vi "WaveGenerator_Sample_Program.vi"(0 "System no.":i32=1 min=1 max=4 step=1, 1 "Stop refnum":refnum<vi>, 2 "Affected axis":string="1", 3 "Selection":T1, 4 "DDL":bool, 5 "error in":errorcluster, 6 "Sine Parameters:":T3={"Xo (Start)"=0, "SIN_P Parameters"={"C"=200.0, "A"=10.0, "O"=0.0}, "N (Length)"=500, "Append? (&)"=FALSE} {"N (Length)" min=0 max=1000 step=1; "SIN_P Parameters"."O" format="%.6f"; "SIN_P Parameters"."A" format="%.6f"; "SIN_P Parameters"."C" format="%.6f"}, 7 "Ramp Parameters:":T2={"Xo (Start)"=0, "RAMP Parameters"={"C"=200.0, "J"=0.0, "A"=8.0, "O"=0.0}, "N (Length)"=500, "Append? (&)"=FALSE} {"N (Length)" min=0 max=1000 step=1; "RAMP Parameters"."O" format="%.6f"; "RAMP Parameters"."A" format="%.6f"; "RAMP Parameters"."J" format="%.6f"; "RAMP Parameters"."C" format="%.6f"}, 8 "Start position":dbl format="%.6f") -> (14 "Waveform":dbl[][](graph) caption="Graph showing the commanded (green) and measured (white) waveform and the position error (red).", 19 "Error out":errorcluster)   [LabVIEW 2009]
doc: "This VI demonstrates how to use the wave generator command VIs. It first moves the affected axis to a given start position. Then it runs in a loop, giving the user the options to write sine wave curve segments or ramps into the controllers wave buffer. Wave storage data points are limited to 1000 points to keep transfer times low. The segment length of one waveform - which normally defines the frequency - is predefined as 500 points in this example. Depending on the value of Append? (&), either the old buffer data is overwritten or the new wave will be appended to memory. Please take into account that you can append at most two waveforms since buffer size is limited to 1000 points as mentioned above. \n\nAdjust the following controls to modify the shape of the waveforms.\nN (Length): Waveform (i.e. the points to be modified) goes from 1 to Length. Datapoints from Length to 500 are filled with value of last wave point.\nXo (Start): Position where the first point of the waveform is located. \nC: Center point of the wave. If C = Length/2 then the wave is symmetrical.\nA: Amplitude of the waveform. F(x) = A*sin(x) + O\nO: Offset of the waveform. F(x) = A*sin(x) + O\nJ: Jerk. Means curvature in the transition to or from standstill.\n\nYou have to stop generator output prior to restarting it with a different parameter set. The Start Gen. and Stop Gen. buttons will enable or disable the wave generator output by sending \"WGO 0\" or \"WGO 1\" for the affected axis. If DDL is enabled \"WGO 65\" will be sent respectively. The red Stop button stops the wave generator output on the specified axis and finishes the loop. Please respect the delays that occur while the controller is processing your commands. This is indicated by the \"Busy?\" indicator. See manual for further details. \n\nIn case of an error a button Clear Error will appear and the control buttons above will be disabled. Pressing this button will clear the error status and enable the control buttons again.\nWith DDL ON you can achieve significantly better position accuracy. Compare the target (green), response (white) and error (red) signals on the graph. Since this is a very sensitive mechanism we recommend starting with low amplitudes and adjusting the parameters with caution. The DDL button works only if the controller supports DDL. Contact PI for information on activation of DDL support.\n\nSee User Manual for details about the use of the wave generator.\n\nRun XXXX_Configuration_Setup (with XXXX being the product number of your PI controller) prior to running this VI.\n\nValid for: E-753"
panel:
  out "Gen. running?":bool
  out "DDL":bool
  in  "Clear Error":bool
  out "Busy?":bool
  out "Controller error":bool
  in  "Stop":bool
  # "Wave generator sample program"
  # "This VI demonstrates how to use the wave generator command VIs. It first moves the affected axis to a given start position. Then it runs in a loop, giving the\nuser the options to write sine wave curve segments or ramps into the controllers wave buffer. Wave storage data points are limited to 1000 points\nto keep transfer times low. The segment length of one waveform is predefined as 500 points in this example. Depending on the value of Append? (&), either\nthe old buffer data is overwritten or the new wave will be appended to memory. You have to stop generator output prior to restarting it with a different\nparameter set. The Start Gen. and Stop Gen. buttons will enable or disable the wave generator output by sending \"WGO 0\" or \"WGO 1\" for the affected axis. \nIf DDL is enabled \"WGO 65\" will be sent respectively. The red Stop button stops the wave generator output on the specified axis and finishes the loop. Please\nrespect the delays that occur while the controller is processing your commands. This is indicated by the \"Busy?\" indicator. See manual for further details. \nRun XXXX_Configuration_Setup (with XXXX being the product number of your PI controller) prior to running this VI."
  # "DDL state"
  # "Stop VI\nand wave\ngenerator\noutput"
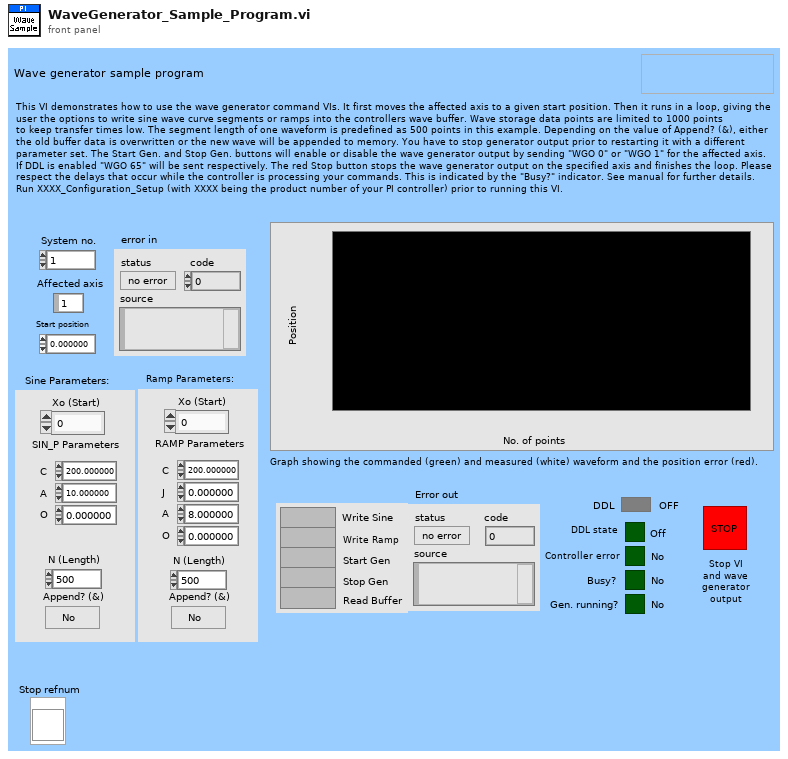
[diagram p1: front panel]
types:
  T1 = cluster{"Write Sine":bool, "Write Ramp":bool, "Start Gen":bool, "Stop Gen":bool, "Read Buffer":bool}
  T2 = cluster{"Xo (Start)":i32, "RAMP Parameters":cluster{"C":dbl, "J":dbl, "A":dbl, "O":dbl}, "N (Length)":i32, "Append? (&)":bool}
  T3 = cluster{"Xo (Start)":i32, "SIN_P Parameters":cluster{"C":dbl, "A":dbl, "O":dbl}, "N (Length)":i32, "Append? (&)":bool}
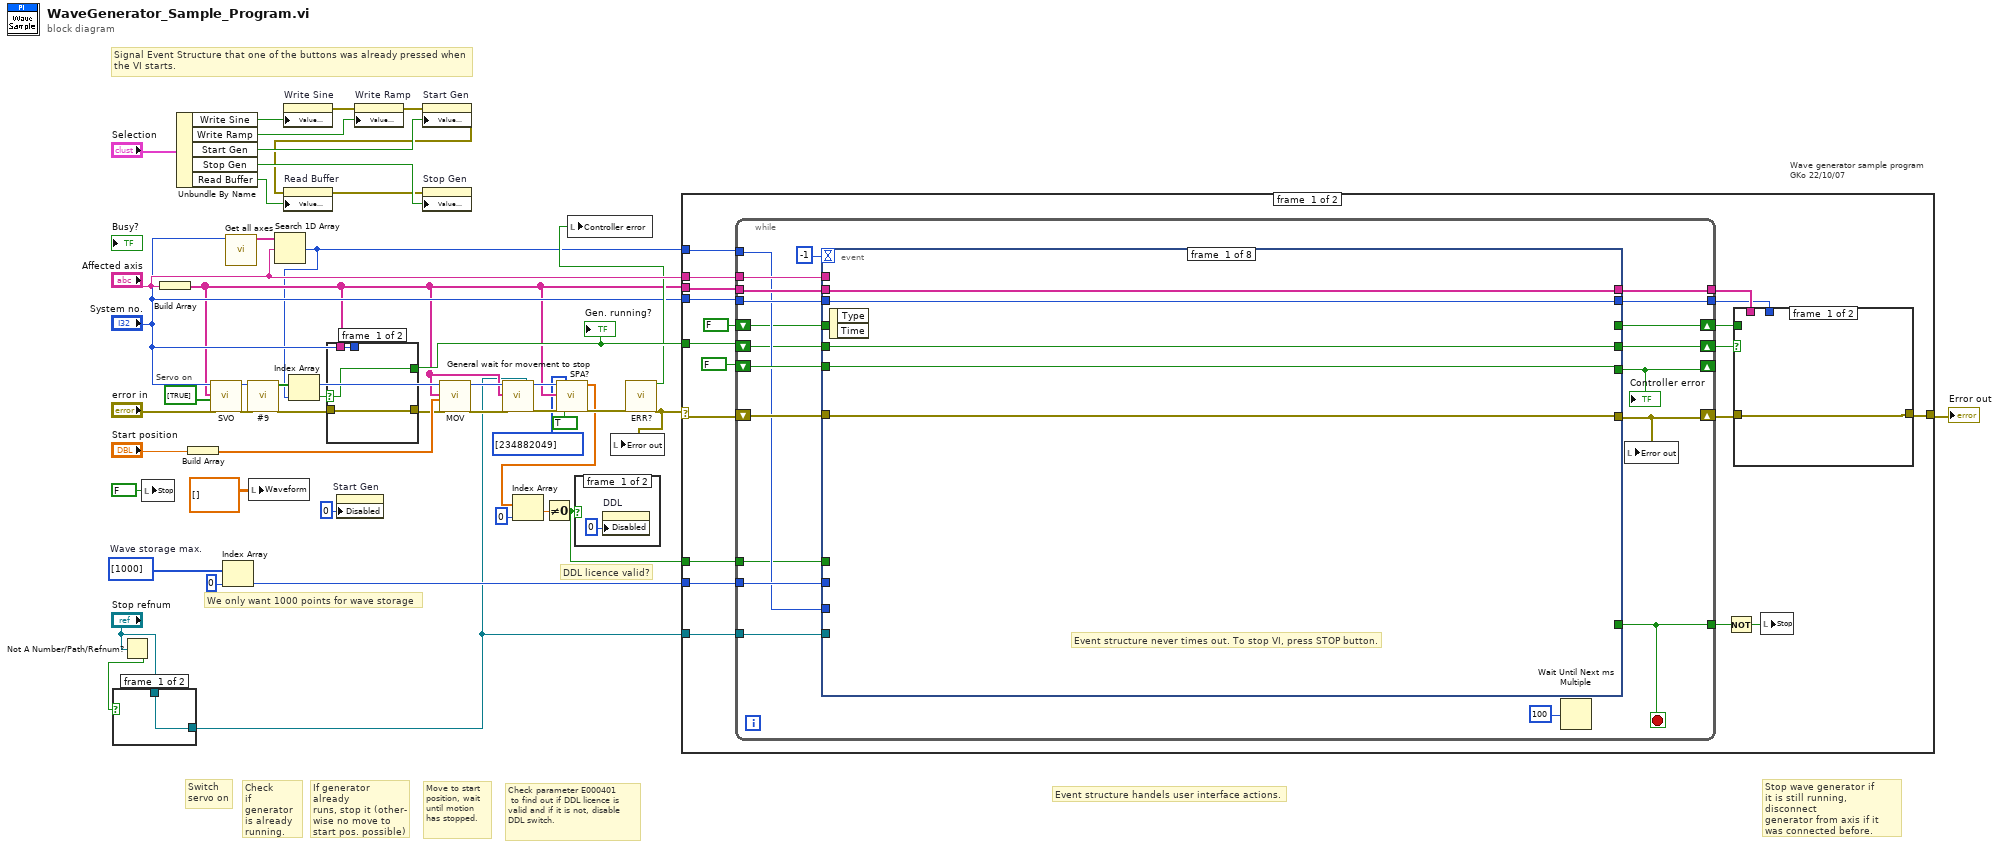
[diagram p0: block diagram]
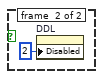
[diagram p2: hidden frame]
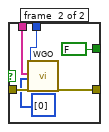
[diagram p3: hidden frame]
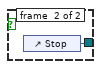
[diagram p4: hidden frame]
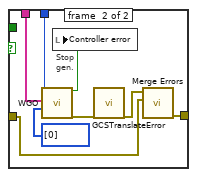
[diagram p5: hidden frame]
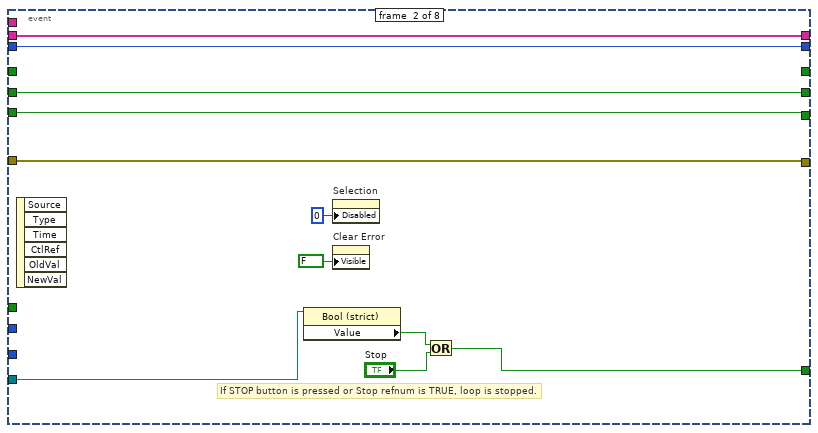
[diagram p6: hidden frame]
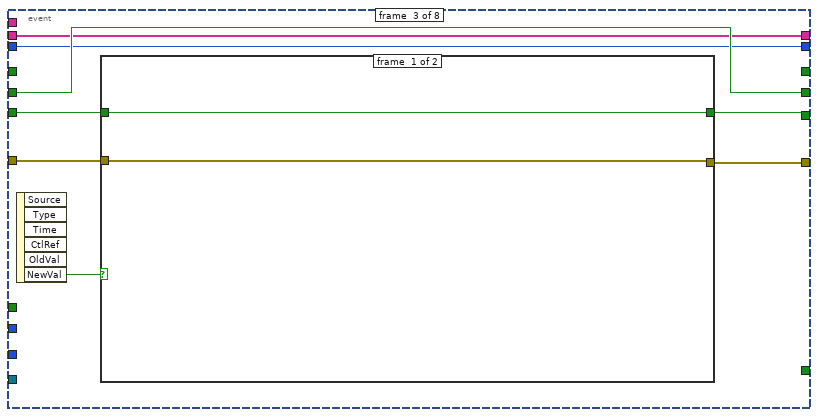
[diagram p7: hidden frame]
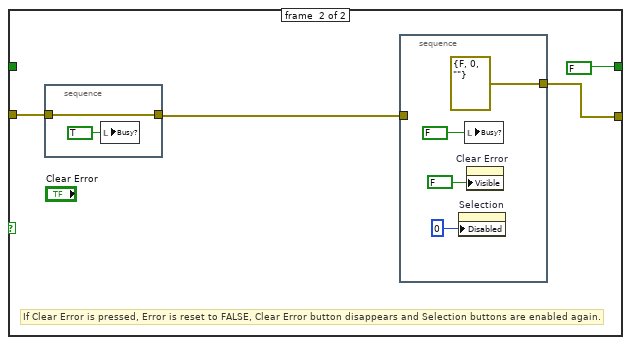
[diagram p8: hidden frame]
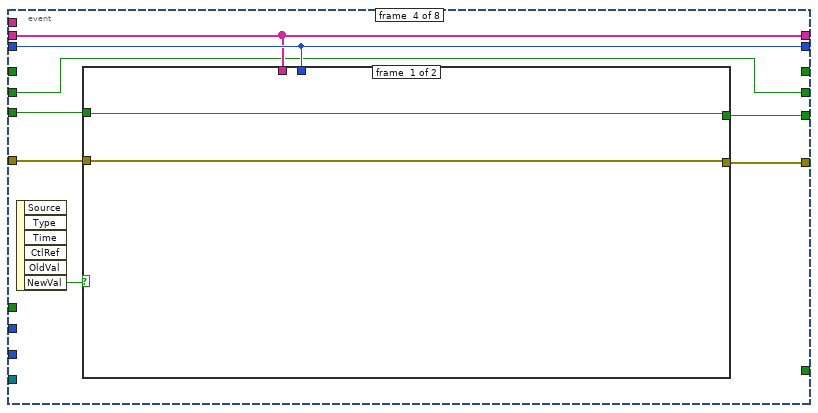
[diagram p9: hidden frame]
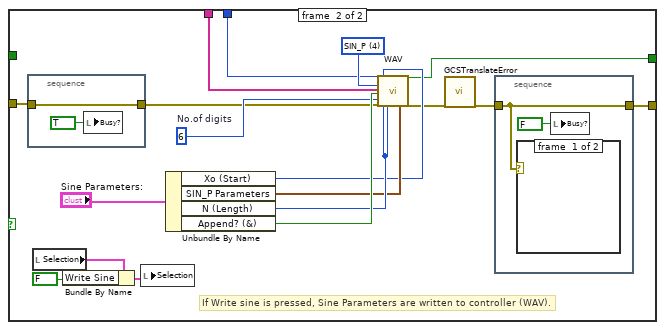
[diagram p10: hidden frame]
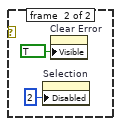
[diagram p11: hidden frame]
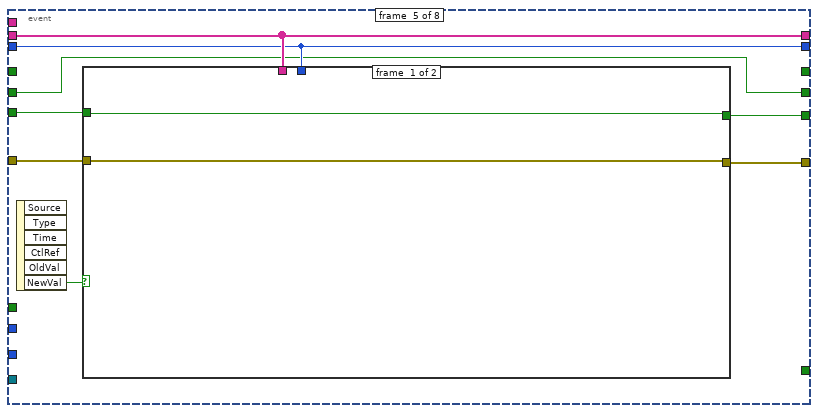
[diagram p12: hidden frame]
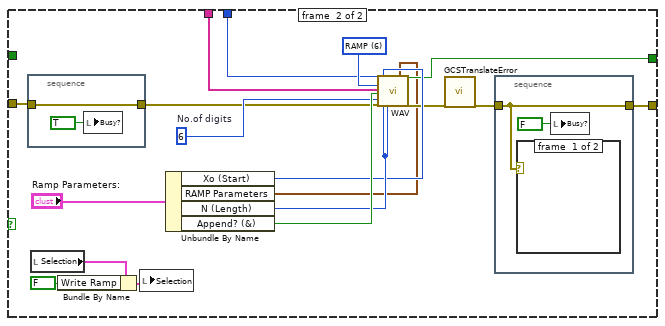
[diagram p13: hidden frame]
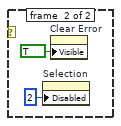
[diagram p14: hidden frame]
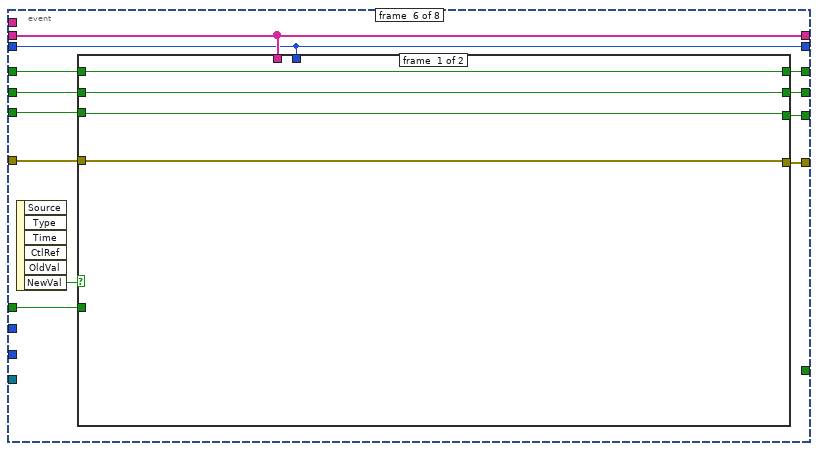
[diagram p15: hidden frame]
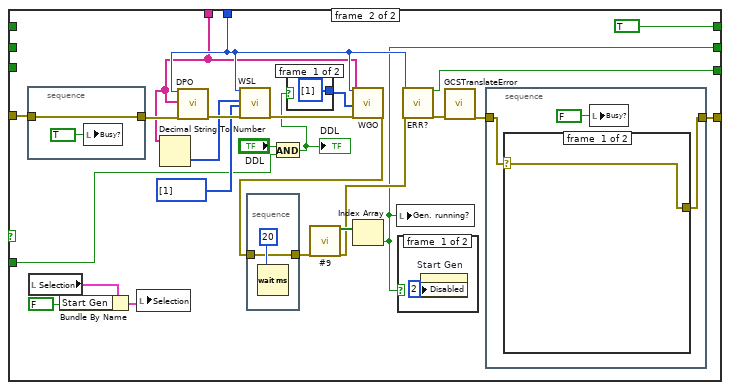
[diagram p16: hidden frame]
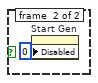
[diagram p17: hidden frame]
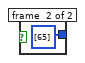
[diagram p18: hidden frame]
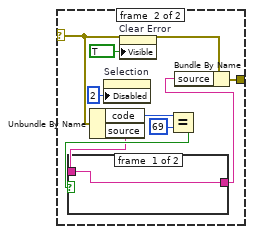
[diagram p19: hidden frame]
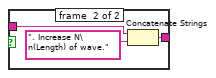
[diagram p20: hidden frame]
diagram:
  w43 = i32[] [1000]  # Wave storage max.
  # "Stop wave generator if\nit is still running, disconnect \ngenerator from axis if it\nwas connected before."
  # "Event structure handels user interface actions."
  # "Check parameter E000401\n to find out if DDL licence is\nvalid and if it is not, disable\nDDL switch."
  # "If generator already\nruns, stop it (other-\nwise no move to\nstart pos. possible)"
  # "Check\nif generator\nis already \nrunning."
  # "We only want 1000 points for wave storage"
  # "Switch\nservo on"
  # "Signal Event Structure that one of the buttons was already pressed when\nthe VI starts."
  # "DDL licence valid?"
  # "Servo on"
  # "Move to start\nposition, wait\nuntil motion\nhas stopped."
  # "Wave generator sample program\nGKo 22/10/07"
  n1 = Not A Number/Path/Refnum?(number/path/refnum="Stop refnum") -> (NaN/Path/Refnum?=w39:bool)
  n2 = case shown="True" w39 {
    tunnel: [w47 w48] -> w5
    tunnel: "Stop refnum" -> [w47 _]
    frame #0 {
    }
    frame #1 {
      n3 = control-ref of="Stop"() -> (w48:refnum<vi>)
    }
  }
  n4 = local write "Stop"(FALSE ("Controller error")) -> ()
  n5 = Build Array("Affected axis") -> (w19:string[])
  n6 = Unbundle By Name("Selection") -> ("Write Sine"=w10:bool, "Write Ramp"=w9:bool, "Start Gen"=w8:bool, "Stop Gen"=w7:bool, "Read Buffer"=w6:bool)
  n7 = Build Array("Start position") -> (w40:dbl[])
  n8 = call "SVO.vi"("System no."="System no.", "Axes to command"=w19, "Servo mode"=bool[] [TRUE], "error in"="error in") -> ("error out"=w33:errorcluster)  [unwired: 15 in]
  n9 = Index Array(array=w43, index=0 ("Index")) -> (element=w44:i32)
  n10 = call "Get all axes.vi"("System no."="System no.") -> ("Conn. Axes"=w35:string[])  [unwired: 18 in]
  n11 = call "#9.vi"("System no."="System no.", "error in"=w33) -> ("WG running?"=w36:bool[], "error out"=w28:errorcluster)  [unwired: 16 in]
  n12 = local write "Waveform"(dbl[][] [] ("Waveform")) -> ()
  n13 = Search 1D Array(1D array=w35, element="Affected axis") -> (index of element=w15:i32)  [unwired: 1 in]
  n14 = property on="Write Sine" class="Boolean (strict)"("Value (Signaling)"=w10) -> (error out=w4:errorcluster)  [unwired: 2 in, 1 out]
  n15 = Index Array(array=w36, index=w15) -> (element=w29:bool)
  n16 = case shown="True" w29 {
    selector: w29 -> [w50 _]
    tunnel: w28 -> [w49 w56]
    tunnel: [w49 w55] -> w27
    tunnel: "System no." -> [_ w53]
    tunnel: w19 -> [_ w52]
    tunnel: [w50 FALSE] -> w26
    frame #0 {
    }
    frame #1 {
      n17 = call "WGO.vi"("System no."=w53, "Affected axes"=w52, "WGO Parameter"=i32[] [0], "error in"=w56) -> ("error out"=w55:errorcluster)  [unwired: 14 in, 1 out]
    }
  }
  "Gen. running?" <- w26
  n18 = property on="Start Gen" class="Bool (strict)"("Disabled"=u8 0) -> ()  [unwired: 2 in, 2 out]
  n19 = property on="Write Ramp" class="Boolean (strict)"(error in=w4, "Value (Signaling)"=w9) -> (error out=w3:errorcluster)  [unwired: 1 in, 1 out]
  n20 = property on="Start Gen" class="Boolean (strict)"(error in=w3, "Value (Signaling)"=w8) -> (error out=w2:errorcluster)  [unwired: 1 in, 1 out]
  n21 = property on="Stop Gen" class="Boolean (strict)"(error in=w2, "Value (Signaling)"=w7) -> (error out=w1:errorcluster)  [unwired: 1 in, 1 out]
  n22 = property on="Read Buffer" class="Boolean (strict)"(error in=w1, "Value (Signaling)"=w6) -> ()  [unwired: 1 in, 2 out]
  n23 = call "MOV.vi"("System no."="System no.", "Axes to move"=w19, "Position values"=w40, "error in"=w27) -> ("error out"=w30:errorcluster)  [unwired: 15 in]
  n24 = call "General wait for movement to stop.vi"("System no."="System no.", "Axes to wait for"=w19, "error in"=w30, "Stop refnum"=w5) -> ("error out"=w21:errorcluster)  [unwired: 14 in, 1 out]
  n25 = call "SPA?.vi"("System no."="System no.", "Axes to query"=w19, "error in"=w21, "Parameter no. (hex)"=u32[] [234882049], "Parameter no. format \n(Decimal: FALSE)"=TRUE ("Parameter no. format \n(Decimal: FALSE)")) -> ("Parameter value"=w16:dbl[], "error out"=w22:errorcluster)  [unwired: 9 in, 4 out]
  n26 = Index Array(array=w16, index=0) -> (element=w13:dbl)
  n27 = Not Equal To 0?(x=w13) -> (x != 0?=w12:bool)
  n28 = case shown="True" w12 {
    frame #0 {
      n29 = property on="DDL" class="Boolean (strict)"("Disabled"=u8 0) -> ()  [unwired: 2 in, 2 out]
    }
    frame #1 {
      n30 = property on="DDL" class="Boolean (strict)"("Disabled"=u8 2) -> ()  [unwired: 2 in, 2 out]
    }
  }
  n31 = call "ERR?.vi"("error in"=w22) -> ("Controller error"=w24:bool, "error out"=w25:errorcluster)  [unwired: 17 in]
  n32 = local write "Controller error"(w24) -> ()
  n33 = local write "Error out"(w25) -> ()
  n34 = case shown="No Error" w25 {
    selector: w25 -> [w69 w372]
    tunnel: w19 -> [w77 _]
    tunnel: "System no." -> [w76 _]
    tunnel: [w67 w371] -> w46
    tunnel: w44 -> [w70 _]
    tunnel: "Affected axis" -> [w72 _]
    tunnel: w15 -> [w68 _]
    tunnel: w26 -> [w66 _]
    tunnel: w12 -> [w60 _]
    tunnel: w5 -> [w59 _]
    frame #0 {
      n35 = while {
        tunnel: w72 -> [w98]
        tunnel: w70 -> [w99]
        shift-left: w69 -> [w101]
        shift-right: [w100] -> w73
        tunnel: [w102] -> w74
        tunnel: [w104] -> w75
        tunnel: w76 -> [w103]
        tunnel: w77 -> [w105]
        shift-right: [w96] -> _
        shift-left: FALSE ("Controller error") -> [w95]
        tunnel: w68 -> [w94]
        shift-right: [w92] -> w65
        shift-left: w66 -> [w93]
        tunnel: [w91] -> w64
        shift-right: [w90] -> w61
        shift-left: FALSE -> [w89]
        tunnel: w60 -> [w88]
        tunnel: w59 -> [w87]
        stop <- w91 stop-if-true
        n36 = event shown="[4] \"Selection.Write Ramp\": Value Change" {
          selector: _ -> [_ _ _ _ _ _ _ _]
          dyn-events: _ -> [_ _ _ _ _ _ _ _]
          timeout: -1 -> [_ _ _ _ _ _ _ _]
          tunnel: w105 -> [w109 w120 w123 w144 w179 w217 w280 w319]
          tunnel: [w109 w120 w123 w144 w179 w217 w280 w319] -> w104
          tunnel: w103 -> [w108 w119 w124 w145 w178 w216 w279 w320]
          tunnel: [w108 w119 w124 w145 w178 w216 w279 w320] -> w102
          tunnel: w101 -> [w110 w121 w126 w148 w182 w220 w284 w326]
          tunnel: [w110 w121 w127 w149 w183 w221 w285 w327] -> w100
          tunnel: w99 -> [_ _ _ _ _ _ _ w321]
          tunnel: w98 -> [_ _ _ _ _ _ _ w322]
          tunnel: [w111 w122 w128 w150 w184 w222 w286 w328] -> w96
          tunnel: w95 -> [w111 w122 w129 w146 w180 w218 w282 w324]
          tunnel: w94 -> [_ _ _ _ _ _ w281 w323]
          tunnel: [_ w114 _ _ _ _ _ _] -> w91
          tunnel: w93 -> [w107 w118 w125 w143 w177 w214 w277 w318]
          tunnel: [w107 w118 w125 w143 w177 w215 w278 w318] -> w92
          tunnel: [_ _ _ _ _ w213 _ _] -> w90
          tunnel: w89 -> [_ _ _ _ _ w212 _ _]
          tunnel: w88 -> [_ _ _ _ _ w211 _ _]
          tunnel: w87 -> [_ w117 _ _ _ _ _ _]
          event #0 {
            # "Event structure never times out. To stop VI, press STOP button."
            n37 = event-data() -> ()  [unwired: 1 in, 2 out]
          }
          event #1 {
            # "If STOP button is pressed or Stop refnum is TRUE, loop is stopped."
            n38 = event-data() -> ()  [unwired: 1 in, 6 out]
            n39 = property class="Bool (strict)"(reference=w117) -> ("Value"=w116:bool)  [unwired: 1 in, 2 out]
            n40 = property on="Selection" class="Cluster (strict)"("Disabled"=u8 0) -> ()  [unwired: 2 in, 2 out]
            n41 = property on="Clear Error" class="Boolean"("Visible"=FALSE) -> ()  [unwired: 2 in, 2 out]
            n42 = Or(x=w116, y="Stop") -> (x .or. y?=w114:bool)
          }
          event #2 {
            n43 = event-data() -> ("NewVal"=w130:bool)  [unwired: 1 in, 5 out]
            n44 = case shown="True" w130 {
              tunnel: w129 -> [w132 _]
              tunnel: [w132 FALSE ("Controller error")] -> w128
              tunnel: [w131 w134] -> w127
              tunnel: w126 -> [w131 w135]
              frame #0 {
              }
              frame #1 {
                # "If Clear Error is pressed, Error is reset to FALSE, Clear Error button disappears and Selection buttons are enabled again."
                n45 = stacked-sequence {
                  tunnel: w135 -> [w141]
                  tunnel: [w141] -> w133
                  frame #0 {
                    n46 = local write "Busy?"(TRUE) -> ()
                  }
                }
                n47 = stacked-sequence {
                  tunnel: [errorcluster {"status"=FALSE, "code"=0, "source"=""} ("error IO")] -> w134
                  tunnel: w133 -> [_]
                  frame #0 {
                    n48 = property on="Selection" class="Clust (strict)"("Disabled"=u8 0) -> ()  [unwired: 2 in, 2 out]
                    n49 = local write "Busy?"(FALSE) -> ()
                    n50 = property on="Clear Error" class="Boolean"("Visible"=FALSE) -> ()  [unwired: 2 in, 2 out]
                  }
                }
              }
            }
          }
          event #3 {
            n51 = event-data() -> ("NewVal"=w147:bool)  [unwired: 1 in, 5 out]
            n52 = case shown="True" w147 {
              tunnel: [w151 w163] -> w150
              tunnel: w145 -> [_ w155]
              tunnel: w144 -> [_ w154]
              tunnel: [w152 w160] -> w149
              tunnel: w148 -> [w152 w159]
              tunnel: w146 -> [w151 _]
              frame #0 {
              }
              frame #1 {
                w166 = i16 6  # No.of digits
                w165 = u16 4 items=["SIN", "POL", "TAN", "PNT", "SIN_P", "LIN", "RAMP"] ("Waveform")
                # "If Write sine is pressed, Sine Parameters are written to controller (WAV)."
                n53 = stacked-sequence {
                  tunnel: w159 -> [w171]
                  tunnel: [w171] -> w153
                  frame #0 {
                    n54 = local write "Busy?"(TRUE) -> ()
                  }
                }
                n55 = local read "Selection"() -> (w158:T1)
                n56 = Bundle By Name(cluster=w158, "Write Sine"=FALSE) -> (w157:T1)
                n57 = local write "Selection"(w157) -> ()
                n58 = Unbundle By Name("Sine Parameters:") -> ("Xo (Start)"=w167:i32, "SIN_P Parameters"=w168:cluster{"C":dbl, "A":dbl, "O":dbl}, "N (Length)"=w169:i32, "Append? (&)"=w170:bool)
                n59 = call "WAV.vi"("System no."=w155, "Waveform"=w165, "Affected axes"=w154, "Append? (&)"=w170, "No.of digits"=w166, "error in"=w153, "Xo"=w167, "N"=w169, "Segment length"=w169, "SIN_P Parameters"=w168) -> ("Controller error"=w163:bool, "error out"=w162:errorcluster)  [unwired: 16 in]
                n60 = call "GCSTranslateError.vi"("error in"=w162) -> ("error out"=w161:errorcluster)  [unwired: 16 in, 2 out]
                n61 = stacked-sequence {
                  tunnel: w161 -> [w173]
                  tunnel: [w173] -> w160
                  frame #0 {
                    n62 = case shown="Error" w173 {
                      frame #0 {
                      }
                      frame #1 {
                        n63 = property on="Selection" class="Clust (strict)"("Disabled"=u8 2) -> ()  [unwired: 2 in, 2 out]
                        n64 = property on="Clear Error" class="Boolean"("Visible"=TRUE) -> ()  [unwired: 2 in, 2 out]
                      }
                    }
                    n65 = local write "Busy?"(FALSE) -> ()
                  }
                }
              }
            }
          }
          event #4 {
            n66 = event-data() -> ("NewVal"=w181:bool)  [unwired: 1 in, 5 out]
            n67 = case shown="True" w181 {
              tunnel: [w185 w199] -> w184
              tunnel: w178 -> [_ w198]
              tunnel: w179 -> [_ w197]
              tunnel: [w186 w194] -> w183
              tunnel: w182 -> [w186 w193]
              tunnel: w180 -> [w185 _]
              frame #0 {
              }
              frame #1 {
                w201 = i16 6  # No.of digits
                w200 = u16 6 items=["SIN", "POL", "TAN", "PNT", "SIN_P", "LIN", "RAMP"] ("Waveform")
                n68 = stacked-sequence {
                  tunnel: w193 -> [w205]
                  tunnel: [w205] -> w192
                  frame #0 {
                    n69 = local write "Busy?"(TRUE) -> ()
                  }
                }
                n70 = local read "Selection"() -> (w189:T1)
                n71 = Bundle By Name(cluster=w189, "Write Ramp"=FALSE ("Write Sine")) -> (w188:T1)
                n72 = local write "Selection"(w188) -> ()
                n73 = Unbundle By Name("Ramp Parameters:") -> ("Xo (Start)"=w202:i32, "RAMP Parameters"=w190:cluster{"C":dbl, "J":dbl, "A":dbl, "O":dbl}, "N (Length)"=w203:i32, "Append? (&)"=w204:bool)
                n74 = call "WAV.vi"("System no."=w198, "Waveform"=w200, "Affected axes"=w197, "Append? (&)"=w204, "No.of digits"=w201, "error in"=w192, "Xo"=w202, "N"=w203, "Segment length"=w203, "RAMP Parameters"=w190) -> ("Controller error"=w199:bool, "error out"=w196:errorcluster)  [unwired: 16 in]
                n75 = call "GCSTranslateError.vi"("error in"=w196) -> ("error out"=w195:errorcluster)  [unwired: 16 in, 2 out]
                n76 = stacked-sequence {
                  tunnel: w195 -> [w207]
                  tunnel: [w207] -> w194
                  frame #0 {
                    n77 = case shown="Error" w207 {
                      frame #0 {
                      }
                      frame #1 {
                        n78 = property on="Selection" class="Clust (strict)"("Disabled"=u8 2) -> ()  [unwired: 2 in, 2 out]
                        n79 = property on="Clear Error" class="Boolean"("Visible"=TRUE) -> ()  [unwired: 2 in, 2 out]
                      }
                    }
                    n80 = local write "Busy?"(FALSE) -> ()
                  }
                }
              }
            }
          }
          event #5 {
            n81 = event-data() -> ("NewVal"=w219:bool)  [unwired: 1 in, 5 out]
            n82 = case shown="True" w219 {
              tunnel: [w225 w241] -> w222
              tunnel: w216 -> [_ w240]
              tunnel: w217 -> [_ w239]
              tunnel: [w226 w250] -> w221
              tunnel: w220 -> [w226 w249]
              tunnel: w218 -> [w225 _]
              tunnel: [w224 w234] -> w215
              tunnel: w214 -> [w224 _]
              tunnel: [w223 TRUE] -> w213
              tunnel: w212 -> [w223 _]
              tunnel: w211 -> [_ w228]
              frame #0 {
              }
              frame #1 {
                n83 = stacked-sequence {
                  tunnel: w249 -> [w258]
                  tunnel: [w258] -> w243
                  frame #0 {
                    n84 = local write "Busy?"(TRUE) -> ()
                  }
                }
                n85 = local read "Selection"() -> (w233:T1)
                n86 = Bundle By Name(cluster=w233, "Start Gen"=FALSE ("Write Sine")) -> (w232:T1)
                n87 = local write "Selection"(w232) -> ()
                n88 = Decimal String To Number(string=w239) -> (number=w244:i32[])  [unwired: 2 in, 1 out]
                n89 = call "DPO.vi"("System no."=w240, "DPO axes"=w239, "error in"=w243) -> ("error out"=w246:errorcluster)  [unwired: 16 in]
                n90 = call "WSL.vi"("System no."=w240, "Generator ID"=w244, "WaveTableID"=i32[] [1], "error in"=w246) -> ("error out"=w247:errorcluster)  [unwired: 15 in]
                n91 = And(x="DDL", y=w228) -> (x .and. y?=w227:bool)
                "DDL" <- w227
                n92 = case shown="True" w227 {
                  tunnel: [i32[] [1] ("WGO Parameter") i32[] [65] ("WGO Parameter")] -> w248
                  frame #0 {
                  }
                  frame #1 {
                  }
                }
                n93 = call "WGO.vi"("System no."=w240, "Affected axes"=w239, "WGO Parameter"=w248, "error in"=w247) -> ("error out"=w236:errorcluster)  [unwired: 14 in, 1 out]
                n94 = stacked-sequence {
                  tunnel: w236 -> [w254]
                  tunnel: [w254] -> w238
                  frame #0 {
                    n95 = Wait (ms)(milliseconds to wait=u32 20) -> ()  [unwired: 1 out]
                  }
                }
                n96 = call "#9.vi"("error in"=w238) -> ("WG running?"=w237:bool[], "error out"=w235:errorcluster)  [unwired: 17 in]
                n97 = Index Array(array=w237) -> (element=w234:bool)  [unwired: 1 in]
                n98 = local write "Gen. running?"(w234) -> ()
                n99 = case shown="True" w234 {
                  frame #0 {
                    n100 = property on="Start Gen" class="Bool (strict)"("Disabled"=u8 2) -> ()  [unwired: 2 in, 2 out]
                  }
                  frame #1 {
                    n101 = property on="Start Gen" class="Bool (strict)"("Disabled"=u8 0) -> ()  [unwired: 2 in, 2 out]
                  }
                }
                n102 = call "ERR?.vi"("System no."=w240, "error in"=w235) -> ("Controller error"=w241:bool, "error out"=w242:errorcluster)  [unwired: 16 in]
                n103 = call "GCSTranslateError.vi"("error in"=w242) -> ("error out"=w251:errorcluster)  [unwired: 16 in, 2 out]
                n104 = stacked-sequence {
                  tunnel: w251 -> [w261]
                  tunnel: [w260] -> w250
                  frame #0 {
                    n105 = case shown="Error" w261 {
                      selector: w261 -> [w263 w268]
                      tunnel: [w263 w266] -> w260
                      frame #0 {
                      }
                      frame #1 {
                        n106 = Unbundle By Name(w268) -> ("code"=w270:i32, "source"=w264:string)
                        n107 = property on="Selection" class="Clust (strict)"("Disabled"=u8 2) -> ()  [unwired: 2 in, 2 out]
                        n108 = property on="Clear Error" class="Boolean"("Visible"=TRUE) -> ()  [unwired: 2 in, 2 out]
                        n109 = Equal?(x=w270, y=69) -> (x = y?=w265:bool)
                        n110 = case shown="True" w265 {
                          tunnel: [w273 w275] -> w267
                          tunnel: w264 -> [w273 w274]
                          frame #0 {
                          }
                          frame #1 {
                            n111 = Concatenate Strings(w274, ". Increase N\n(Length) of wave.") -> (w275:string)
                          }
                        }
                        n112 = Bundle By Name(cluster=w268, "source"=w267) -> (w266:errorcluster)
                      }
                    }
                    n113 = local write "Busy?"(FALSE) -> ()
                  }
                }
              }
            }
          }
          event #6 {
            n114 = event-data() -> ("NewVal"=w283:bool)  [unwired: 1 in, 5 out]
            n115 = case shown="True" w283 {
              tunnel: [w288 w302] -> w286
              tunnel: w279 -> [_ w296]
              tunnel: w280 -> [_ w301]
              tunnel: [w289 w306] -> w285
              tunnel: w284 -> [w289 w305]
              tunnel: w282 -> [w288 _]
              tunnel: w281 -> [_ w294]
              tunnel: [w287 w293] -> w278
              tunnel: w277 -> [w287 _]
              frame #0 {
              }
              frame #1 {
                n116 = stacked-sequence {
                  tunnel: w305 -> [w312]
                  tunnel: [w312] -> w300
                  frame #0 {
                    n117 = local write "Busy?"(TRUE) -> ()
                  }
                }
                n118 = local read "Selection"() -> (w292:T1)
                n119 = Bundle By Name(cluster=w292, "Stop Gen"=FALSE ("Write Sine")) -> (w291:T1)
                n120 = local write "Selection"(w291) -> ()
                n121 = call "WGO.vi"("System no."=w296, "Affected axes"=w301, "WGO Parameter"=i32[] [0], "error in"=w300) -> ("error out"=w299:errorcluster)  [unwired: 14 in, 1 out]
                n122 = stacked-sequence {
                  tunnel: w299 -> [w310]
                  tunnel: [w310] -> w298
                  frame #0 {
                    n123 = Wait (ms)(milliseconds to wait=u32 20) -> ()  [unwired: 1 out]
                  }
                }
                n124 = call "#9.vi"("System no."=w296, "error in"=w298) -> ("WG running?"=w295:bool[], "error out"=w297:errorcluster)  [unwired: 16 in]
                n125 = Index Array(array=w295, index=w294) -> (element=w293:bool)
                n126 = local write "Gen. running?"(w293) -> ()
                n127 = case shown="True" w293 {
                  frame #0 {
                    n128 = property on="Start Gen" class="Bool (strict)"("Disabled"=u8 2) -> ()  [unwired: 2 in, 2 out]
                  }
                  frame #1 {
                    n129 = property on="Start Gen" class="Bool (strict)"("Disabled"=u8 0) -> ()  [unwired: 2 in, 2 out]
                  }
                }
                n130 = call "ERR?.vi"("System no."=w296, "error in"=w297) -> ("Controller error"=w302:bool, "error out"=w303:errorcluster)  [unwired: 16 in]
                n131 = call "GCSTranslateError.vi"("error in"=w303) -> ("error out"=w307:errorcluster)  [unwired: 16 in, 2 out]
                n132 = stacked-sequence {
                  tunnel: w307 -> [w314]
                  tunnel: [w314] -> w306
                  frame #0 {
                    n133 = case shown="Error" w314 {
                      frame #0 {
                      }
                      frame #1 {
                        n134 = property on="Selection" class="Clust (strict)"("Disabled"=u8 2) -> ()  [unwired: 2 in, 2 out]
                        n135 = property on="Clear Error" class="Boolean"("Visible"=TRUE) -> ()  [unwired: 2 in, 2 out]
                      }
                    }
                    n136 = local write "Busy?"(FALSE) -> ()
                  }
                }
              }
            }
          }
          event #7 {
            n137 = event-data() -> ("NewVal"=w325:bool)  [unwired: 1 in, 5 out]
            n138 = case shown="True" w325 {
              tunnel: [w329 w340] -> w328
              tunnel: w320 -> [_ w337]
              tunnel: w319 -> [_ _]
              tunnel: [w330 w363] -> w327
              tunnel: w326 -> [w330 w362]
              tunnel: w324 -> [w329 _]
              tunnel: w323 -> [_ _]
              tunnel: w322 -> [_ w336]
              tunnel: w321 -> [_ w334]
              frame #0 {
              }
              frame #1 {
                w348 = 3 ("Numeric")
                w349 = 2 ("Numeric")
                w356 = 1 ("Numeric")
                # "Record and display values"
                n139 = stacked-sequence {
                  tunnel: w362 -> [w365]
                  tunnel: [w365] -> w338
                  frame #0 {
                    n140 = local write "Busy?"(TRUE) -> ()
                  }
                }
                n141 = call "DRC.vi"("System no."=w337, "Rec. table"=w356, "Rec. option"=w356, "error in"=w338, "Source ID"=w336) -> ("Controller error"=w346:bool, "error out"=w355:errorcluster)  [unwired: 13 in]
                n142 = call "DRC.vi"("System no."=w337, "Rec. table"=w349, "Rec. option"=w349, "error in"=w355, "Source ID"=w336) -> ("Controller error"=w345:bool, "error out"=w354:errorcluster)  [unwired: 13 in]
                n143 = call "DRC.vi"("System no."=w337, "Rec. table"=w348, "Rec. option"=w348, "error in"=w354, "Source ID"=w336) -> ("Controller error"=w344:bool, "error out"=w347:errorcluster)  [unwired: 13 in]
                n144 = call "WGR.vi"("System no."=w337, "error in"=w347) -> ("error out"=w342:errorcluster)  [unwired: 17 in]
                n145 = call "DRR?.vi"("System no."=w337, "Rec. table IDs"=i32[] [1, 2, 3], "error in"=w342, "Xo"=1, "N"=w334, "Nmax"=w334) -> ("Data"=w359:dbl[][], "error out"=w339:errorcluster)  [unwired: 10 in, 2 out]
                n146 = Index Array(array=w359, index (col) #1=0 ("Disabled Index (col)"), index (col) #2=1 ("Disabled Index (col)"), index (col) #3=2 ("Disabled Index (col)")) -> (element #1=w357:dbl[], element #2=w351:dbl[], element #3=w350:dbl[])  [unwired: 3 in]
                n147 = Build Array(w357, w351, w350) -> (→"Waveform":dbl[][])
                n148 = call "ERR?.vi"("System no."=w337, "error in"=w339) -> ("Controller error"=w341:bool, "error out"=w361:errorcluster)  [unwired: 16 in]
                n149 = call "GCSTranslateError.vi"("error in"=w361) -> ("error out"=w364:errorcluster)  [unwired: 16 in, 2 out]
                n150 = Compound Arithmetic op=OR(w341, w346, w345, w344) -> (w340:bool)
                n151 = stacked-sequence {
                  tunnel: w364 -> [w367]
                  tunnel: [w367] -> w363
                  frame #0 {
                    n152 = case shown="Error" w367 {
                      frame #0 {
                      }
                      frame #1 {
                        n153 = property on="Selection" class="Clust (strict)"("Disabled"=u8 2) -> ()  [unwired: 2 in, 2 out]
                        n154 = property on="Clear Error" class="Boolean"("Visible"=TRUE) -> ()  [unwired: 2 in, 2 out]
                      }
                    }
                    n155 = local write "Busy?"(FALSE) -> ()
                  }
                }
                n156 = local read "Selection"() -> (w333:T1)
                n157 = Bundle By Name(cluster=w333, "Read Buffer"=FALSE ("Write Sine")) -> (w332:T1)
                n158 = local write "Selection"(w332) -> ()
              }
            }
          }
        }
        "Controller error" <- w96
        n159 = Wait Until Next ms Multiple(millisecond multiple=u32 100) -> ()  [unwired: 1 out]
        n160 = local write "Error out"(w100) -> ()
      }
      n161 = Not(x=w64) -> (.not. x?=w63:bool)
      n162 = case shown="True" w65 {
        tunnel: w75 -> [_ w83]
        tunnel: w74 -> [_ w84]
        tunnel: w73 -> [w78 w80]
        tunnel: [w78 w82] -> w67
        tunnel: w61 -> [_ _]
        frame #0 {
        }
        frame #1 {
          # "Stop\ngen."
          n163 = call "WGO.vi"("System no."=w84, "Affected axes"=w83, "WGO Parameter"=i32[] [0] ("WGO \nParameter")) -> ("Controller error"=w85:bool, "error out"=w79:errorcluster)  [unwired: 15 in]
          n164 = local write "Controller error"(w85) -> ()
          n165 = call "GCSTranslateError.vi"("error in"=w79) -> ("error out"=w81:errorcluster)  [unwired: 16 in, 2 out]
          n166 = call <vilib>:"Merge Errors.vi"("error in 2 (no error)"=w80, "error in 1 (no error)"=w81) -> ("error out"=w82:errorcluster)  [unwired: 5 in]
        }
      }
      n167 = local write "Stop"(w63) -> ()
    }
    frame #1 {
      n168 = call "GCSTranslateError.vi"("error in"=w372) -> ("error out"=w371:errorcluster)  [unwired: 16 in, 2 out]
    }
  }
  "Error out" <- w46
